vi "AlliGator Get Simulation Parameters (by x Factor).vi"(6 "Use Experimental IRF":bool, 8 "Simulation Parameters x Factor":T4, 9 "Fit Simulation Parameters":T3, 10 "Decay Simulation Parameters":T2, 11 "# Steps":i32) -> (3 "Simulation Parameters Array":T1[](array[typedef]))   [LabVIEW 2021, in "AlliGator Fit Method Benchmark.lvlib"]
uses:
  AlliGator Fit Method Benchmark.lvlib
  AlliGator Simulation Parameters x Factors.ctl
  AlliGator Fit Simulation Parameters.ctl
  AlliGator Decay Simulation Parameters.ctl
  AlliGator Simulation Parameters.ctl
panel:
  # "see the License on the block diagram (Ctrl+E or Window:Show Block Diagram)"
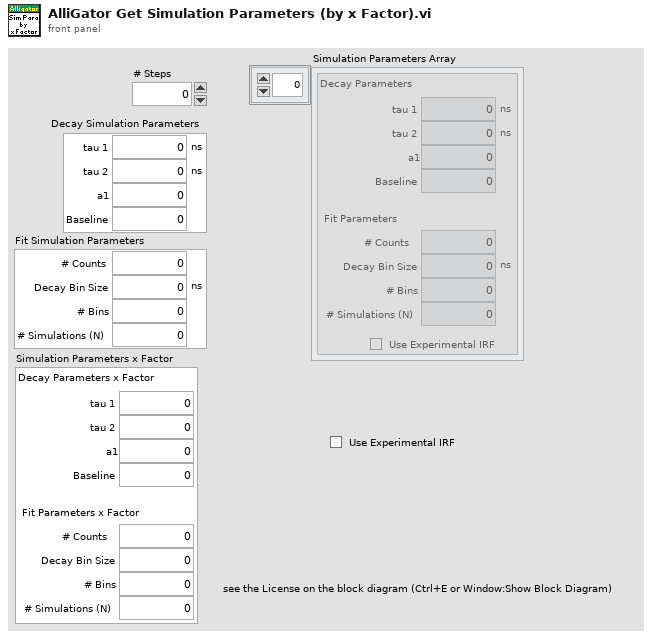
[diagram p1: front panel]
types:
  T1 = typedef "AlliGator Fit Method Benchmark.lvlib/AlliGator Simulation Parameters.ctl" = cluster{"Decay Simulation Parameters":T2, "Fit Simulation Parameters":T3, "Use Experimental IRF":bool}
  T2 = typedef "AlliGator Fit Method Benchmark.lvlib/AlliGator Decay Simulation Parameters.ctl" = cluster{"tau 1":dbl[unit], "tau 2":dbl[unit], "a1":dbl, "Baseline":dbl}
  T3 = typedef "AlliGator Fit Method Benchmark.lvlib/AlliGator Fit Simulation Parameters.ctl" = cluster{"# Counts":i32, "# Simulations (N)":i32, "Decay Bin Size":dbl[unit], "# Bins":i32}
  T4 = typedef "AlliGator Fit Method Benchmark.lvlib/AlliGator Simulation Parameters x Factors.ctl" = cluster{"Decay Simulation Parameters":cluster{"tau 1":dbl, "tau 2":dbl, "a1":dbl, "Baseline":dbl}, "Fit Simulation Parameters":cluster{"# Counts":dbl, "# Simulations (N)":dbl, "Decay Bin Size":dbl, "# Bins":dbl}}
  T5 = cluster{"# Counts":dbl, "# Simulations (N)":dbl, "Decay Bin Size":dbl, "# Bins":dbl}
  T6 = cluster{"tau 1":dbl, "tau 2":dbl, "a1":dbl, "Baseline":dbl}
  T7 = cluster{"# Counts":dbl, "# Simulations (N)":dbl, "Decay Bin Size":dbl[unit], "# Bins":dbl}
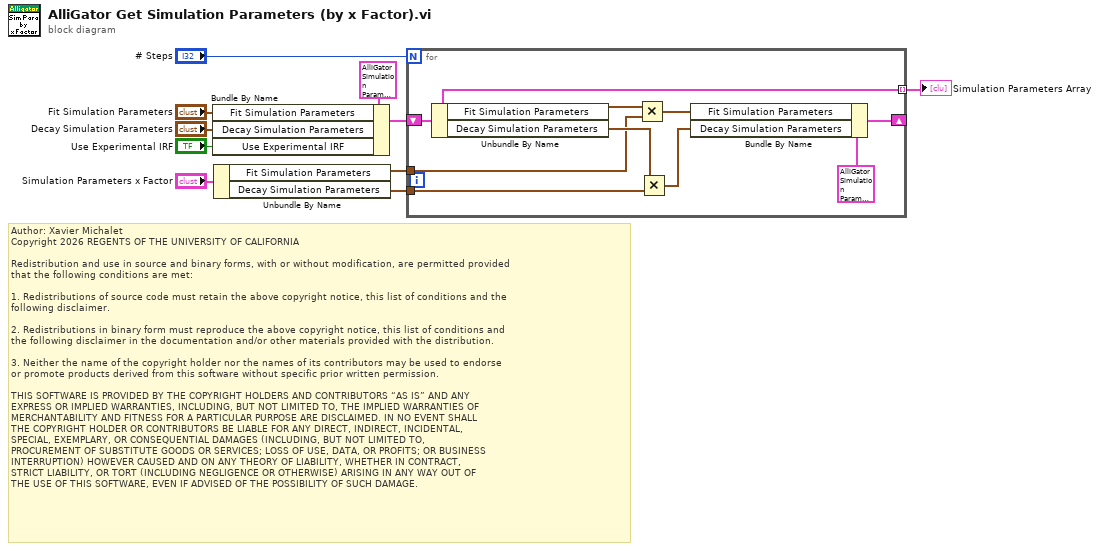
[diagram p0: block diagram]
diagram:
  # "Author: Xavier Michalet\nCopyright 2026 REGENTS OF THE UNIVERSITY OF CALIFORNIA\n\nRedistribution and use in source and binary forms, with or without modification, are permitted provided\nthat the following conditions are met:\n\n1. Redistributions of source code must retain the above copyright notice, this list of conditions and the\nfollowing disclaimer.\n\n2. Redistributions in binary form must reproduce the above copyright notice, this list of conditions and\nthe following disclaimer in the documentation and/or other materials provided with the distribution.\n\n3. Neither the name of the copyright holder nor the names of its contributors may be used to endorse \nor promote products derived from this software without specific prior written permission.\n\nTHIS SOFTWARE IS PROVIDED BY THE COPYRIGHT HOLDERS AND CONTRIBUTORS “AS IS” AND ANY \nEXPRESS OR IMPLIED WARRANTIES, INCLUDING, BUT NOT LIMITED TO, THE IMPLIED WARRANTIES OF\nMERCHANTABILITY AND FITNESS FOR A PARTICULAR PURPOSE ARE DISCLAIMED. IN NO EVENT SHALL\nTHE COPYRIGHT HOLDER OR CONTRIBUTORS BE LIABLE FOR ANY DIRECT, INDIRECT, INCIDENTAL, \nSPECIAL, EXEMPLARY, OR CONSEQUENTIAL DAMAGES (INCLUDING, BUT NOT LIMITED TO, \nPROCUREMENT OF SUBSTITUTE GOODS OR SERVICES; LOSS OF USE, DATA, OR PROFITS; OR BUSINESS\nINTERRUPTION) HOWEVER CAUSED AND ON ANY THEORY OF LIABILITY, WHETHER IN CONTRACT, \nSTRICT LIABILITY, OR TORT (INCLUDING NEGLIGENCE OR OTHERWISE) ARISING IN ANY WAY OUT OF\nTHE USE OF THIS SOFTWARE, EVEN IF ADVISED OF THE POSSIBILITY OF SUCH DAMAGE."
  n1 = Bundle By Name(cluster=T1 {"Decay Simulation Parameters"={"tau 1"=1e-09, "tau 2"=0.0, "a1"=1.0, "Baseline"=0.0}, "Fit Simulation Parameters"={"# Counts"=100, "# Simulations (N)"=100, "Decay Bin Size"=1.0000000000000002e-10, "# Bins"=200}, "Use Experimental IRF"=FALSE} ("Simulation Parameters Array"), "Fit Simulation Parameters"="Fit Simulation Parameters", "Decay Simulation Parameters"="Decay Simulation Parameters", "Use Experimental IRF"="Use Experimental IRF") -> (w6:T1)
  n2 = Unbundle By Name("Simulation Parameters x Factor") -> ("Fit Simulation Parameters"=w3:T5, "Decay Simulation Parameters"=w2:T6)
  n3 = for {
    N: "# Steps" -> [_]
    shift-right: [w18] -> _
    shift-left: w6 -> [w13]
    tunnel: [w13] -> w5 mode=indexing
    tunnel: w3 -> [w12]
    tunnel: w2 -> [w11]
    n4 = Unbundle By Name(w13) -> ("Fit Simulation Parameters"=w15:T3, "Decay Simulation Parameters"=w14:T2)
    n5 = Multiply(x=w15, y=w12) -> (x*y=w19:T7)
    n6 = Multiply(x=w14, y=w11) -> (x*y=w17:T2)
    n7 = Bundle By Name(cluster=T1 {"Decay Simulation Parameters"={"tau 1"=1e-09, "tau 2"=0.0, "a1"=1.0, "Baseline"=0.0}, "Fit Simulation Parameters"={"# Counts"=100, "# Simulations (N)"=100, "Decay Bin Size"=1.0000000000000002e-10, "# Bins"=200}, "Use Experimental IRF"=FALSE} ("Simulation Parameters Array"), "Fit Simulation Parameters"=w19, "Decay Simulation Parameters"=w17) -> (w18:T1)
  }
  "Simulation Parameters Array" <- w5
